vi "start.vi"(7 "LabVIEW Web Service Request":refnum<class "Web Request.lvclass">) -> ()   [LabVIEW 2019]
uses:
  <vilib>/wsapi/Web Request.lvclass
  Controls/Test Action.ctl
panel:
  # "Use the Web Service Request input terminal to call the VIs on the Web Services palette. Do not remove it from the connector pane unless you don't need access to the palette."
  # "Each additional control wired to the connector pane will be available as an input in the URL. To include an indicator in terminal-mode output (the default setting), it must also be wired to the connector pane."
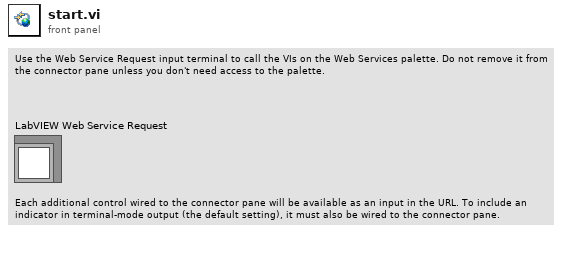
[diagram p1: front panel]
types:
  T1 = typedef "Test Action.ctl" = enum16{"Idle", "Start", "Stop", "Pump Cmd", "Pump 1 Enable", "Pump 2 Enable", "Pump 3 Enable", "Pump 4 Enable", "Pump 5 Enable", "Pump 6 Enable", "Timer 1 Reset", "Timer 2 Reset", "Timer 3 Reset", "Timer 4 Reset", "Timer 5 Reset", "Timer 6 Reset"}
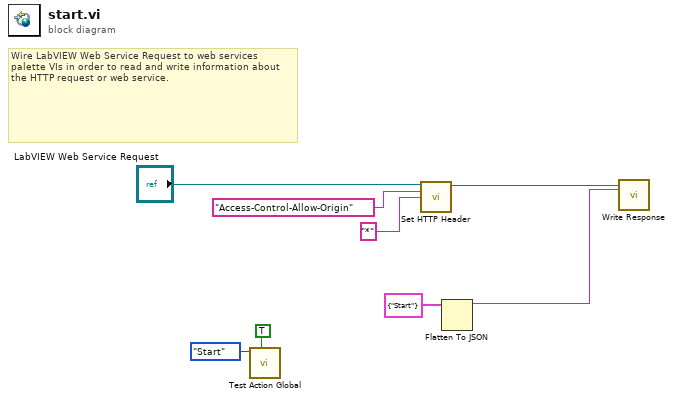
[diagram p0: block diagram]
diagram:
  # "Wire LabVIEW Web Service Request to web services palette VIs in order to read and write information about the HTTP request or web service."
  n1 = call "Test Action Global.vi"("Write (F)"=TRUE, "Test Action IN"=Test_Action."Start") -> ()  [unwired: 8 in, 2 out]
  n2 = call <vilib>:"Set HTTP Header.vi"("LabVIEW Web Service Request"="LabVIEW Web Service Request", "header"="Access-Control-Allow-Origin" ("header value"), "header value"="*" ("header")) -> ("LabVIEW Web Service Request out"=w7:refnum<class "Web Request.lvclass">)  [unwired: 11 in, 1 out]
  n3 = Flatten To JSON(anything=cluster{"Action":string} {"Action"="Start"}) -> (JSON string=w4:string)  [unwired: 2 in, 1 out]
  n4 = call <vilib>:"Write Response.vi"("LabVIEW Web Service Request"=w7, "response string"=w4) -> ()  [unwired: 12 in, 2 out]
